vi "Parse MEGA.vi"(10 "path":path) -> (2 "MEGA Traj":T9(array[cluster]) {"?"."Overrides"."Angle Override" step=5.0; "?"."Overrides"."Velocity Override" step=5.0; "?"."Overrides"."Angular Override" step=5.0; "?"."Angular Limits"."Jerk (deg/s^3)" min=0.0 step=1.0; "?"."Angular Limits"."Accel (deg/s^2)" min=0.0; "?"."Angular Limits"."Velocity (deg/s)" min=0.0})   [LabVIEW 2023]
uses:
  Types/Trajectory Data.ctl
  Types/Segment Type.ctl
  Types/Single Cmd Info.ctl
  <vilib>/picture/picture.llb/imagedata.ctl
  Types/Overrides.ctl
  Types/Angluar Limits.ctl
  Types/Drive Type.ctl
  Types/Path Type.ctl
  Types/Availible Command systems for auto.ctl
  Types/Limits.ctl
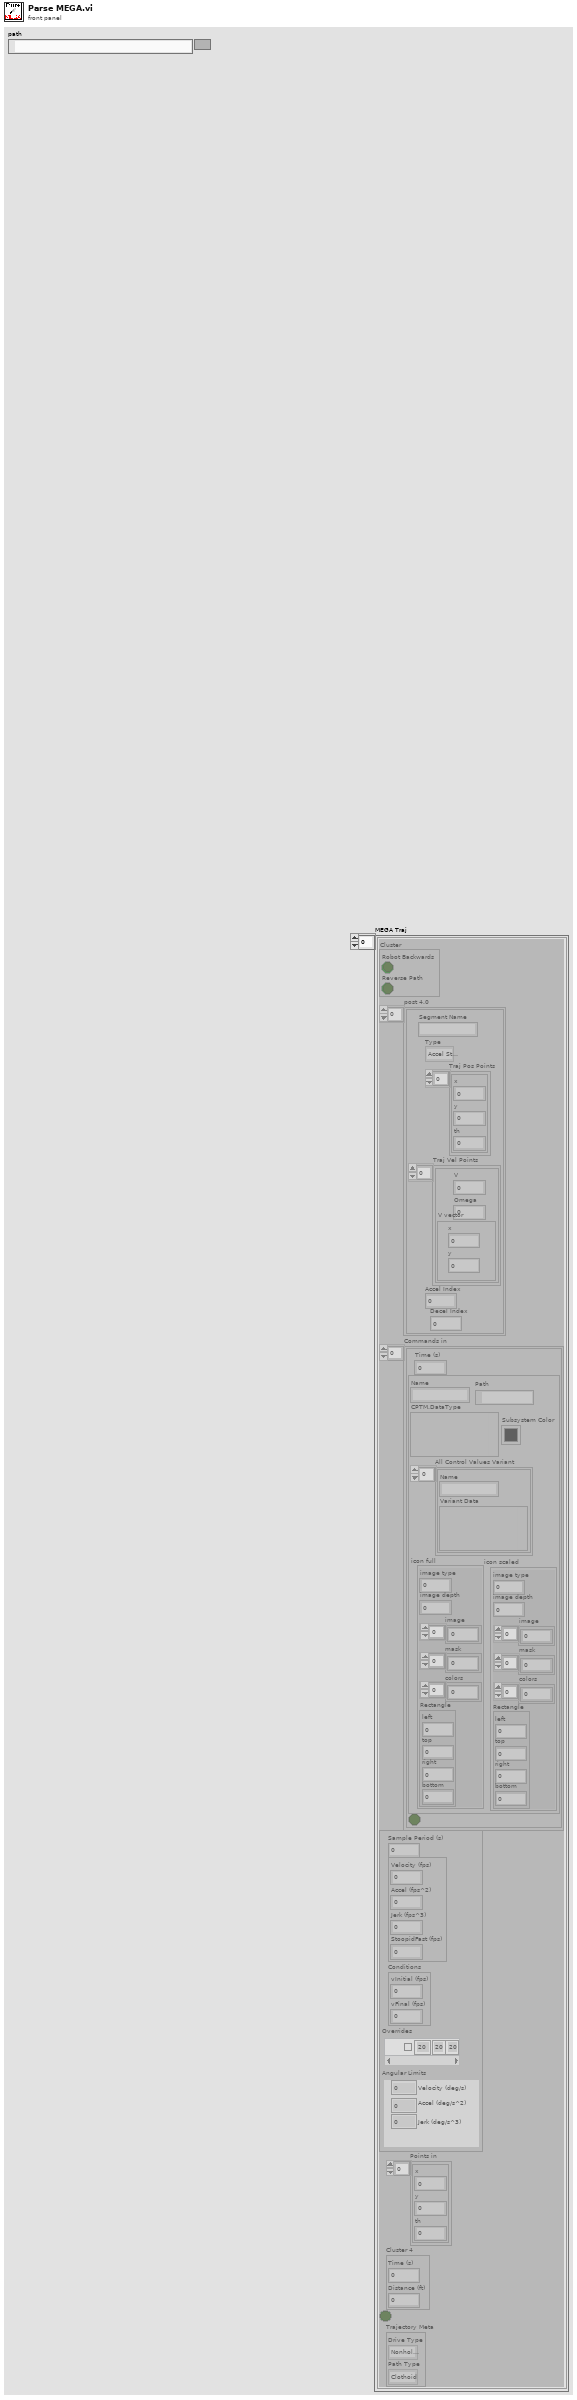
[diagram p1: front panel]
types:
  T1 = typedef "Trajectory Data.ctl" = cluster{"Segment Name":string, "Type":T2, "Traj Pos Points":cluster{"x":dbl, "y":dbl, "th":dbl}[], "Traj Vel Points":cluster{"V":dbl, "Omega":dbl, "V vector":cluster{"y":dbl, "x":dbl}}[], "Accel Index":i32, "Decel Index":i32}[]
  T2 = typedef "Segment Type.ctl" = enum16{"Accel Straight", "Const Straight", "Blend", "Circle", "Bezier"}
  T3 = typedef "Single Cmd Info.ctl" = cluster{"Name":string, "CPTM.DataType":variant, "All Control Values Variant":cluster{"Name":string, "Variant Data":variant}[], "icon full":T4, "icon scaled":T4, "Path":path, "Subsystem Color":u32}
  T4 = typedef "imagedata.ctl" = cluster{"image type":i32, "image depth":i32, "image":u8[], "mask":u8[], "colors":u32[], "Rectangle":cluster{"left":i16, "top":i16, "right":i16, "bottom":i16}}
  T5 = typedef "Overrides.ctl" = cluster{"Count":string, "Angular Override":dbl, "Enabled?":bool, "Velocity Override":dbl, "Angle Override":dbl}[]
  T6 = typedef "Angluar Limits.ctl" = cluster{"Velocity (deg/s)":dbl, "Accel (deg/s^2)":dbl, "Jerk (deg/s^3)":dbl}
  T7 = typedef "Drive Type.ctl" = enum16{"Nonholonomic", "Holonomic"}
  T8 = typedef "Path Type.ctl" = enum16{"Clothoid", "Bezier"}
  T9 = cluster{"Cluster":cluster{"Robot Backwards":bool, "Reverse Path":bool}, "post 4.0":T1, "Commands in":cluster{"Time (s)":dbl, T3, bool}[], cluster{"Sample Period (s)":dbl, cluster{"Velocity (fps)":dbl, "Accel (fps^2)":dbl, "Jerk (fps^3)":dbl, "StoopidFast (fps)":dbl}, "Conditions":cluster{"vInitial (fps)":dbl, "vFinal (fps)":dbl}, "Overrides":T5, "Angular Limits":T6}, "Points in":cluster{"x":dbl, "y":dbl, "th":dbl}[], "Cluster 4":cluster{"Time (s)":dbl, "Distance (ft)":dbl}, bool, "Trajectory Meta":cluster{"Drive Type":T7, "Path Type":T8}}[]
  T10 = cluster{"Segment Name":string, "Type":T2, "Traj Pos Points":cluster{"x":dbl, "y":dbl, "th":dbl}[], "Traj Vel Points":cluster{"V":dbl, "Omega":dbl}[], "Accel Index":i32, "Decel Index":i32}[]
  T11 = cluster{"Sample Period (s)":dbl, "Limits 2":cluster{"Velocity (fps)":dbl, "Acceleration (fps^2)":dbl, "Jerk (fps^3)":dbl}, "Conditions":cluster{"vInitial (fps)":dbl, "vFinal (fps)":dbl}, " Acceleration Overrides":cluster{"Angular \nAccelerations":dbl[], "Accel Override Bools":bool[]}}
  T12 = cluster{"Velocity":dbl, "Sample Time":dbl, "Accel":dbl}
  T13 = cluster{"Sample Period (s)":dbl, "Limits":cluster{"Velocity (fps)":dbl, "Acceleration (fps^2)":dbl, "Jerk (fps^3)":dbl}, "Conditions":cluster{"vInitial (fps)":dbl, "vFinal (fps)":dbl}}
  T14 = cluster{"Sample Period (s)":dbl, "Limits":cluster{"Velocity (fps)":dbl, "Acceleration (fps^2)":dbl, "Jerk (fps^3)":dbl}, "Conditions":cluster{"vInitial (fps)":dbl, "vFinal (fps)":dbl}, "Min Rads":dbl[]}
  T15 = typedef "Availible Command systems for auto.ctl" = u16
  T16 = cluster{"Time into Path":dbl, "System":T15, "Item Selected?":bool, "System Selection":T15}[]
  T17 = cluster{"Sample Period (s)":dbl, "Limits 2":cluster{"Velocity (fps)":dbl, "Acceleration (fps^2)":dbl, "Jerk (fps^3)":dbl, "Stoopid Fast":dbl}, "Conditions":cluster{"vInitial (fps)":dbl, "vFinal (fps)":dbl}, " Acceleration Overrides":cluster{"Angular \nAccelerations":dbl[], "Accel Override Bools":bool[]}}
  T18 = cluster{"Sample Period (s)":dbl, "Limits":cluster{"Velocity (fps)":dbl, "Accel (fps^2)":dbl, "Turn Accel (fps^2)":dbl, "Jerk (fps^3)":dbl}, "Conditions":cluster{"vInitial (fps)":dbl, "vFinal (fps)":dbl}, cluster{dbl[], bool[]}}
  T19 = cluster{"Reverse Path":bool, "Robot Backwards":bool}
  T20 = cluster{"Robot Backwards":bool, "Reverse Path":bool}
  T21 = typedef "Limits.ctl" = cluster{"Velocity (fps)":dbl, "Accel (fps^2)":dbl, "Jerk (fps^3)":dbl, "StoopidFast (fps)":dbl}
  T22 = cluster{"Sample Period (s)":dbl, "Limits":T21, "Conditions":cluster{"vInitial (fps)":dbl, "vFinal (fps)":dbl}, "Overrides":T5, "Angular Limits":T6}
  T23 = cluster{"Velocity":dbl, "Accel":dbl, "Accel":dbl, "Velocity":dbl}
  T24 = cluster{"Velocity (fps)":dbl, "Acceleration (fps^2)":dbl, "Jerk (fps^3)":dbl}
  T25 = cluster{"vInitial (fps)":dbl, "vFinal (fps)":dbl}
  T26 = cluster{"Velocity (fps)":dbl, "Acceleration (fps^2)":dbl, "Jerk (fps^3)":dbl, "Velocity (fps)":dbl}
  T27 = cluster{string, "Angular Multiplier":dbl, bool, "Velocity (fps)":dbl, "Velocity (fps)":dbl}
  T28 = cluster{"Angular \nAccelerations":dbl[], "Accel Override Bools":bool[]}
  T29 = cluster{"Velocity (fps)":dbl, "Acceleration (fps^2)":dbl, "Jerk (fps^3)":dbl, "Stoopid Fast":dbl}
  T30 = cluster{"Velocity (fps)":dbl, "Accel (fps^2)":dbl, "Turn Accel (fps^2)":dbl, "Jerk (fps^3)":dbl}
  T31 = cluster{"Velocity (fps)":dbl, "Accel (fps^2)":dbl, "Jerk (fps^3)":dbl, "StoopidFast (fps)":dbl}
  T32 = cluster{"Sample Period (s)":dbl, cluster{"Velocity (fps)":dbl, "Accel (fps^2)":dbl, "Jerk (fps^3)":dbl, "StoopidFast (fps)":dbl}, "Conditions":cluster{"vInitial (fps)":dbl, "vFinal (fps)":dbl}, "Overrides":T5, "Angular Limits":T6}
  T33 = cluster{"Cluster":cluster{"Robot Backwards":bool, "Reverse Path":bool}, "post 4.0":T1, "Commands in":cluster{"Time (s)":dbl, T3, bool}[], cluster{"Sample Period (s)":dbl, cluster{"Velocity (fps)":dbl, "Accel (fps^2)":dbl, "Jerk (fps^3)":dbl, "StoopidFast (fps)":dbl}, "Conditions":cluster{"vInitial (fps)":dbl, "vFinal (fps)":dbl}, "Overrides":T5, "Angular Limits":T6}, "Points in":cluster{"x":dbl, "y":dbl, "th":dbl}[], "Cluster 4":cluster{"Time (s)":dbl, "Distance (ft)":dbl}, bool, "Trajectory Meta":cluster{"Drive Type":T7, "Path Type":T8}}
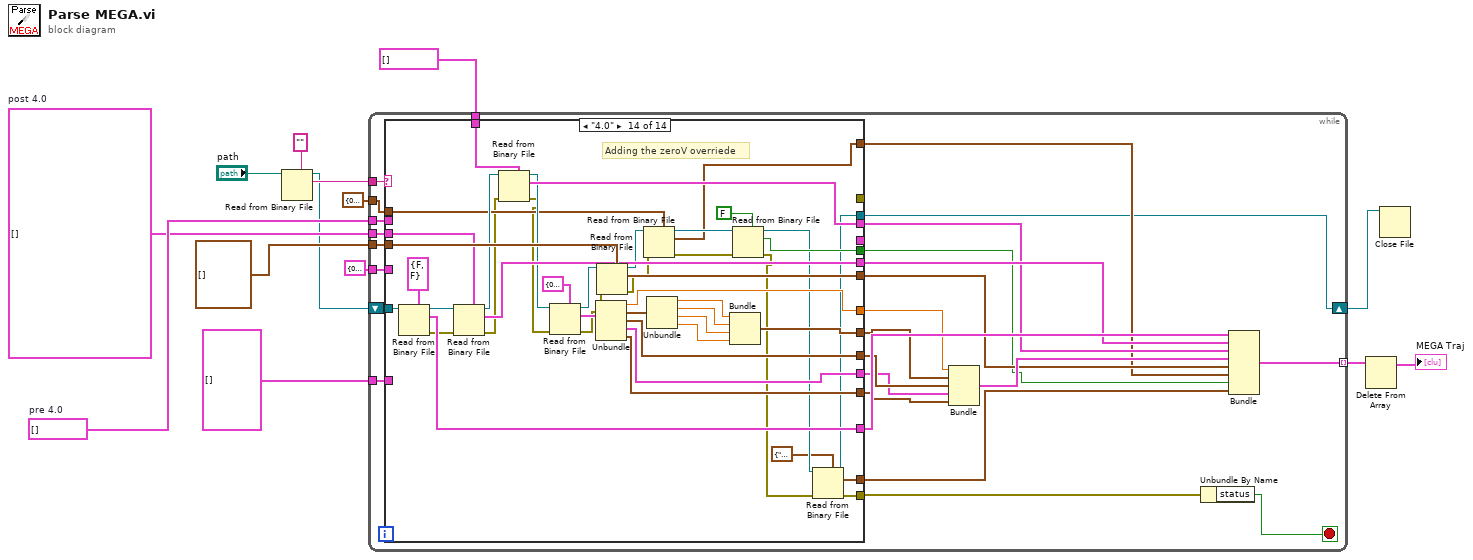
[diagram p0: block diagram]
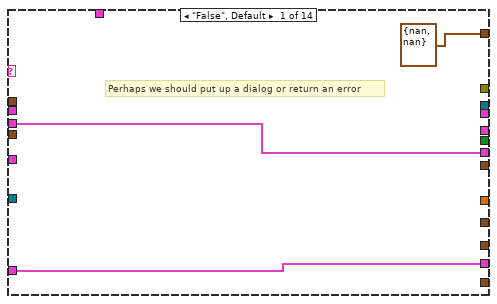
[diagram p2: hidden frame]
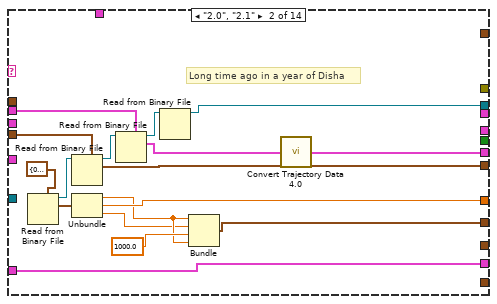
[diagram p3: hidden frame]
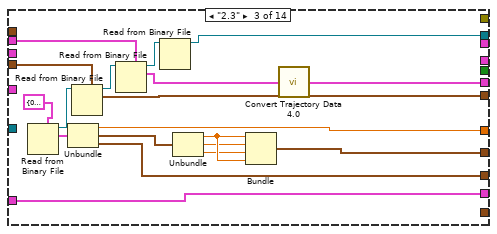
[diagram p4: hidden frame]
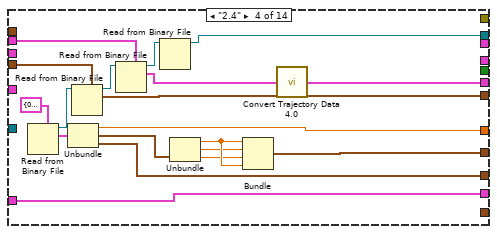
[diagram p5: hidden frame]
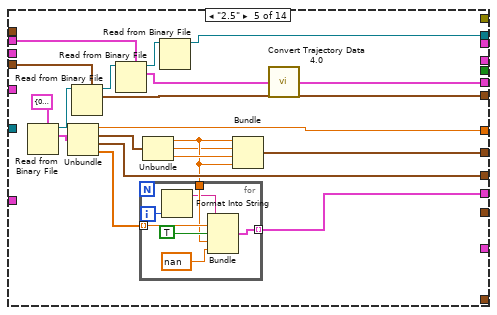
[diagram p6: hidden frame]
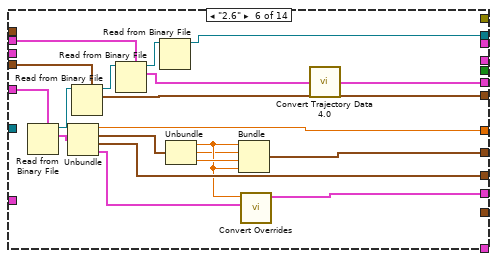
[diagram p7: hidden frame]
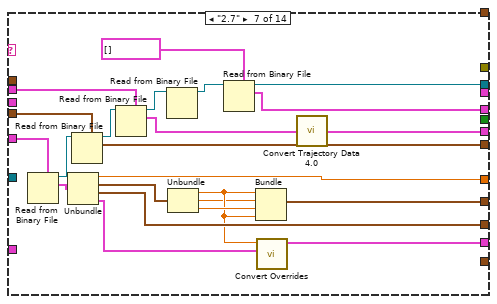
[diagram p8: hidden frame]
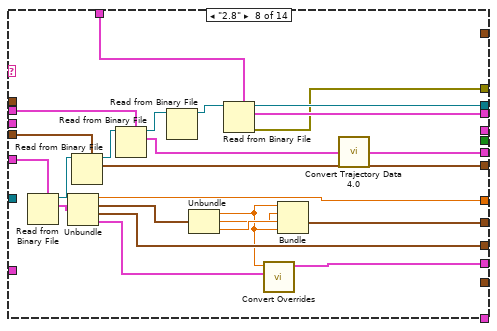
[diagram p9: hidden frame]
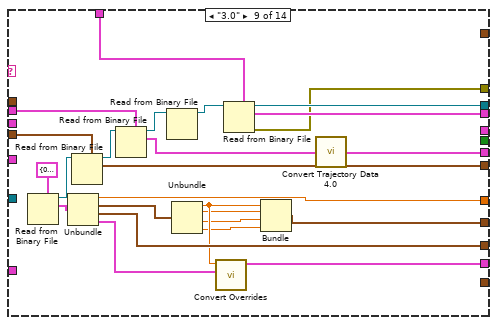
[diagram p10: hidden frame]
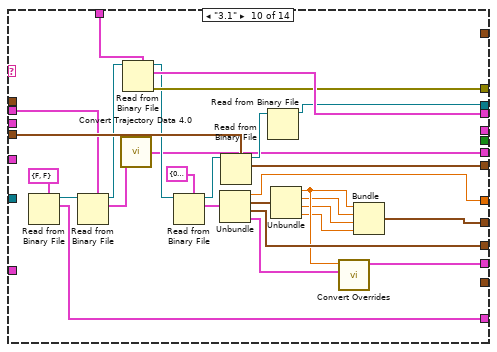
[diagram p11: hidden frame]
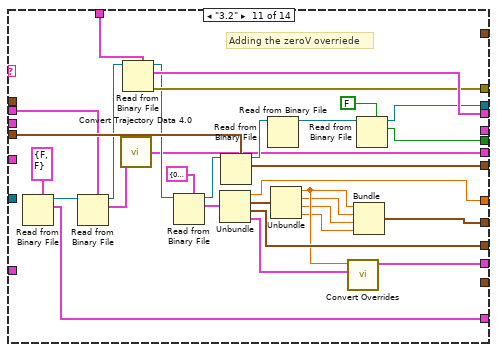
[diagram p12: hidden frame]
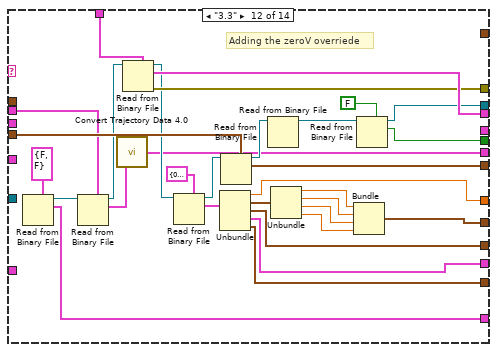
[diagram p13: hidden frame]
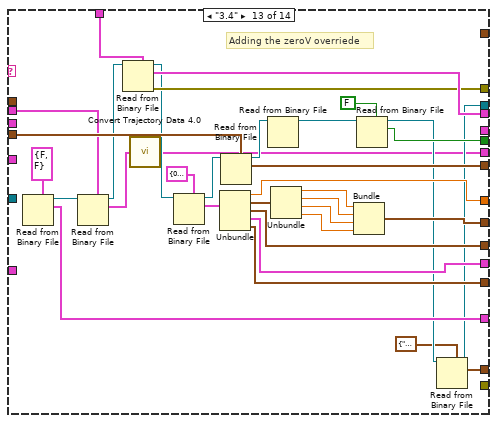
[diagram p14: hidden frame]
diagram:
  w7 = T10 []  # pre 4.0
  w6 = T1 []  # post 4.0
  n1 = Read from Binary File(5:"" ("String"), 11:"path") -> (2:w10:string, 3:w5:refnum<file>)  [unwired: 4 in, 2 out]
  n2 = while {
    tunnel: T11 {"Sample Period (s)"=0.0, "Limits 2"={"Velocity (fps)"=0.0, "Acceleration (fps^2)"=0.0, "Jerk (fps^3)"=0.0}, "Conditions"={"vInitial (fps)"=0.0, "vFinal (fps)"=0.0}, " Acceleration Overrides"={"Angular \nAccelerations"=[], "Accel Override Bools"=[]}} ("Cluster") -> [w40]
    tunnel: cluster{"Time (s)":dbl, T3, bool}[] [] ("Commands in") -> [w39]
    tunnel: cluster{"x":dbl, "y":dbl, "th":dbl}[] [] ("Points in") -> [w38]
    tunnel: w10 -> [w37]
    tunnel: T5 [] ("Overrides") -> [w36]
    tunnel: w7 -> [w35]
    tunnel: w6 -> [w34]
    tunnel: [w20] -> w2 mode=indexing
    tunnel: cluster{"Time (s)":dbl, "Distance (ft)":dbl} {"Time (s)"=0.0, "Distance (ft)"=0.0} ("Cluster 4") -> [w18]
    shift-right: [w16] -> w3
    shift-left: w5 -> [w19]
    stop <- w17 stop-if-true
    n3 = case shown="\"4.0\"" w37 {
      tunnel: w38 -> [_ w58 w77 w96 w116 w143 w166 w190 w215 w243 w274 w305 w339 w382]
      tunnel: [_ w57 w76 w95 w115 w142 w165 w189 w214 w242 w273 w304 w338 w381] -> w29
      tunnel: w35 -> [_ w56 w75 w94 w114 w141 w164 w188 w213 w241 w272 w303 w337 _]
      tunnel: [_ w53 w72 w91 w111 w138 w157 w181 w206 w232 w249 w283 w310 w355] -> w16
      tunnel: [_ w51 w71 w90 w110 w137 w161 w185 w210 w219 w251 w285 w319 w364] -> w25
      tunnel: [_ w47 w65 w83 w104 w132 w151 w176 w194 w224 w256 w290 w324 w369] -> w24
      tunnel: [_ _ w70 w89 w109 w136 w160 w184 w209 w240 w271 w302 w336 w380] -> w23
      tunnel: [w43 w46 w64 w82 w103 w130 w148 w173 w200 w228 w260 w279 w314 w359] -> w22
      tunnel: [w41 w44 w61 w80 w99 w126 w146 w169 w193 w218 w246 w277 w308 w379] -> w31
      tunnel: [_ _ _ _ _ _ w156 _ _ _ _ _ _ _] -> _
      tunnel: w39 -> [_ _ _ _ _ _ _ w180 w205 w238 w269 w300 w334 w378]
      tunnel: [_ _ _ _ _ _ _ w179 w204 w237 w268 w299 w333 w377] -> w30
      tunnel: [_ _ _ _ _ _ _ w178 w203 w236 w267 w298 w332 _] -> _
      tunnel: w40 -> [_ _ _ _ _ w134 w154 w174 _ _ _ _ _ _]
      tunnel: [_ _ _ _ _ _ _ _ _ w227 w259 w292 w326 w371] -> w32
      tunnel: w36 -> [w43 w46 w64 w82 _ _ _ _ _ _ _ _ _ _]
      tunnel: [_ _ _ _ _ _ _ _ _ _ w247 w281 w316 w361] -> w27
      tunnel: [cluster{"Time (s)":dbl, "Distance (ft)":dbl} {"Time (s)"=nan, "Distance (ft)"=nan} ("Cluster 4") _ _ _ _ _ _ _ _ _ _ _ _ w350] -> w28
      tunnel: [_ _ _ _ _ _ _ _ _ _ _ w278 w313 w358] -> w21
      tunnel: [_ _ _ _ _ _ _ _ _ _ _ _ w309 w354] -> w26
      tunnel: w34 -> [w41 _ _ _ _ _ _ _ _ _ _ _ _ w353]
      tunnel: w19 -> [_ _ _ _ _ _ _ _ _ _ _ _ _ w352]
      tunnel: w18 -> [_ _ _ _ _ _ _ _ _ _ _ _ _ w351]
      tunnel: [_ _ _ _ _ _ _ _ _ _ _ _ _ w342] -> w15
      frame "False", Default {
        # "Perhaps we should put up a dialog or return an error"
      }
      frame "2.0", "2.1" {
        # "Long time ago in a year of Disha"
        n4 = Read from Binary File(5:T12 {"Velocity"=0.0, "Sample Time"=0.0, "Accel"=0.0}) -> (2:w60:T12, 3:w59:refnum<file>)  [unwired: 5 in, 2 out]
        n5 = Read from Binary File(5:w58, 11:w59) -> (2:w57:cluster{"x":dbl, "y":dbl, "th":dbl}[], 3:w55:refnum<file>)  [unwired: 4 in, 2 out]
        n6 = Unbundle(w60) -> ("Velocity"=w48:dbl, "Sample Time"=w51:dbl, "Accel"=w45:dbl)
        n7 = Read from Binary File(5:w56, 11:w55) -> (2:w49:T10, 3:w54:refnum<file>)  [unwired: 4 in, 2 out]
        n8 = Read from Binary File(11:w54) -> (3:w53:refnum<file>)  [unwired: 5 in, 3 out]
        n9 = Bundle("Velocity"=w48, "Accel"=w45, "Accel"=1000.0, "Velocity"=w48) -> (w47:T23)  [unwired: 1 in]
        n10 = call "Convert Trajectory Data 4.0.vi"("pre 4.0"=w49) -> ("post 4.0"=w44:T1)
      }
      frame "2.3" {
        n11 = Read from Binary File(5:T13 {"Sample Period (s)"=0.0, "Limits"={"Velocity (fps)"=0.0, "Acceleration (fps^2)"=0.0, "Jerk (fps^3)"=0.0}, "Conditions"={"vInitial (fps)"=0.0, "vFinal (fps)"=0.0}}) -> (2:w79:T13, 3:w78:refnum<file>)  [unwired: 5 in, 2 out]
        n12 = Unbundle(w79) -> ("Sample Period (s)"=w71:dbl, "Limits"=w62:T24, "Conditions"=w70:T25)
        n13 = Read from Binary File(5:w77, 11:w78) -> (2:w76:cluster{"x":dbl, "y":dbl, "th":dbl}[], 3:w74:refnum<file>)  [unwired: 4 in, 2 out]
        n14 = Read from Binary File(5:w75, 11:w74) -> (2:w68:T10, 3:w73:refnum<file>)  [unwired: 4 in, 2 out]
        n15 = Read from Binary File(11:w73) -> (3:w72:refnum<file>)  [unwired: 5 in, 3 out]
        n16 = Unbundle(w62) -> ("Velocity (fps)"=w67:dbl, "Acceleration (fps^2)"=w63:dbl, "Jerk (fps^3)"=w66:dbl)
        n17 = Bundle("Velocity (fps)"=w67, "Acceleration (fps^2)"=w63, "Jerk (fps^3)"=w66, "Velocity (fps)"=w67) -> (w65:T26)  [unwired: 1 in]
        n18 = call "Convert Trajectory Data 4.0.vi"("pre 4.0"=w68) -> ("post 4.0"=w61:T1)
      }
      frame "2.4" {
        n19 = Read from Binary File(5:T13 {"Sample Period (s)"=0.0, "Limits"={"Velocity (fps)"=0.0, "Acceleration (fps^2)"=0.0, "Jerk (fps^3)"=0.0}, "Conditions"={"vInitial (fps)"=0.0, "vFinal (fps)"=0.0}}) -> (2:w98:T13, 3:w97:refnum<file>)  [unwired: 5 in, 2 out]
        n20 = Unbundle(w98) -> ("Sample Period (s)"=w90:dbl, "Limits"=w84:T24, "Conditions"=w89:T25)
        n21 = Read from Binary File(5:w96, 11:w97) -> (2:w95:cluster{"x":dbl, "y":dbl, "th":dbl}[], 3:w93:refnum<file>)  [unwired: 4 in, 2 out]
        n22 = Read from Binary File(5:w94, 11:w93) -> (2:w87:T10, 3:w92:refnum<file>)  [unwired: 4 in, 2 out]
        n23 = Read from Binary File(11:w92) -> (3:w91:refnum<file>)  [unwired: 5 in, 3 out]
        n24 = Unbundle(w84) -> ("Velocity (fps)"=w86:dbl, "Acceleration (fps^2)"=w81:dbl, "Jerk (fps^3)"=w85:dbl)
        n25 = Bundle("Velocity (fps)"=w86, "Acceleration (fps^2)"=w81, "Jerk (fps^3)"=w85, "Velocity (fps)"=w86) -> (w83:T26)  [unwired: 1 in]
        n26 = call "Convert Trajectory Data 4.0.vi"("pre 4.0"=w87) -> ("post 4.0"=w80:T1)
      }
      frame "2.5" {
        n27 = Read from Binary File(5:T14 {"Sample Period (s)"=0.0, "Limits"={"Velocity (fps)"=0.0, "Acceleration (fps^2)"=0.0, "Jerk (fps^3)"=0.0}, "Conditions"={"vInitial (fps)"=0.0, "vFinal (fps)"=0.0}, "Min Rads"=[20.0, 20.0, 20.0, 20.0, 20.0]}) -> (2:w118:T14, 3:w117:refnum<file>)  [unwired: 5 in, 2 out]
        n28 = Unbundle(w118) -> ("Sample Period (s)"=w110:dbl, "Limits"=w105:T24, "Conditions"=w109:T25, "Min Rads"=w102:dbl[])
        n29 = Read from Binary File(5:w116, 11:w117) -> (2:w115:cluster{"x":dbl, "y":dbl, "th":dbl}[], 3:w113:refnum<file>)  [unwired: 4 in, 2 out]
        n30 = Read from Binary File(5:w114, 11:w113) -> (2:w107:T10, 3:w112:refnum<file>)  [unwired: 4 in, 2 out]
        n31 = Unbundle(w105) -> ("Velocity (fps)"=w101:dbl, "Acceleration (fps^2)"=w100:dbl, "Jerk (fps^3)"=w106:dbl)
        n32 = for {
          tunnel: [w124] -> w103 mode=indexing
          tunnel: w102 -> [w123] mode=indexing
          tunnel: w101 -> [w122]
          i -> [w121]
          n33 = Format Into String(w121) -> (resulting string=w120:string)  [unwired: 3 in, 1 out]
          n34 = Bundle(w120, "Angular Multiplier"=w123, TRUE, "Velocity (fps)"=w122, "Velocity (fps)"=nan) -> (w124:T27)  [unwired: 1 in]
        }
        n35 = Read from Binary File(11:w112) -> (3:w111:refnum<file>)  [unwired: 5 in, 3 out]
        n36 = Bundle("Velocity (fps)"=w101, "Acceleration (fps^2)"=w100, "Jerk (fps^3)"=w106, "Velocity (fps)"=w101) -> (w104:T26)  [unwired: 1 in]
        n37 = call "Convert Trajectory Data 4.0.vi"("pre 4.0"=w107) -> ("post 4.0"=w99:T1)
      }
      frame "2.6" {
        n38 = Read from Binary File(5:w134) -> (2:w145:T11, 3:w144:refnum<file>)  [unwired: 5 in, 2 out]
        n39 = Unbundle(w145) -> ("Sample Period (s)"=w137:dbl, "Limits 2"=w131:T24, "Conditions"=w136:T25, "Acceleration Overrides"=w128:T28)
        n40 = Read from Binary File(5:w143, 11:w144) -> (2:w142:cluster{"x":dbl, "y":dbl, "th":dbl}[], 3:w140:refnum<file>)  [unwired: 4 in, 2 out]
        n41 = Read from Binary File(5:w141, 11:w140) -> (2:w135:T10, 3:w139:refnum<file>)  [unwired: 4 in, 2 out]
        n42 = Read from Binary File(11:w139) -> (3:w138:refnum<file>)  [unwired: 5 in, 3 out]
        n43 = Unbundle(w131) -> ("Velocity (fps)"=w129:dbl, "Acceleration (fps^2)"=w127:dbl, "Jerk (fps^3)"=w133:dbl)
        n44 = Bundle("Velocity (fps)"=w129, "Acceleration (fps^2)"=w127, "Jerk (fps^3)"=w133, "Velocity (fps)"=w129) -> (w132:T26)  [unwired: 1 in]
        n45 = call "Convert Overrides.vi"("Cluster"=w128, "Velocity (fps)"=w129) -> ("Overrides"=w130:T5)  [unwired: 9 in]
        n46 = call "Convert Trajectory Data 4.0.vi"("pre 4.0"=w135) -> ("post 4.0"=w126:T1)
      }
      frame "2.7" {
        n47 = Read from Binary File(5:w154) -> (2:w168:T11, 3:w167:refnum<file>)  [unwired: 5 in, 2 out]
        n48 = Unbundle(w168) -> ("Sample Period (s)"=w161:dbl, "Limits 2"=w152:T24, "Conditions"=w160:T25, "Acceleration Overrides"=w149:T28)
        n49 = Read from Binary File(5:w166, 11:w167) -> (2:w165:cluster{"x":dbl, "y":dbl, "th":dbl}[], 3:w163:refnum<file>)  [unwired: 4 in, 2 out]
        n50 = Read from Binary File(5:w164, 11:w163) -> (2:w159:T10, 3:w162:refnum<file>)  [unwired: 4 in, 2 out]
        n51 = Read from Binary File(11:w162) -> (3:w158:refnum<file>)  [unwired: 5 in, 3 out]
        n52 = Unbundle(w152) -> ("Velocity (fps)"=w150:dbl, "Acceleration (fps^2)"=w147:dbl, "Jerk (fps^3)"=w153:dbl)
        n53 = Read from Binary File(5:T16 [] ("Commands"), 11:w158) -> (2:w156:T16, 3:w157:refnum<file>)  [unwired: 4 in, 2 out]
        n54 = Bundle("Velocity (fps)"=w150, "Acceleration (fps^2)"=w147, "Jerk (fps^3)"=w153, "Velocity (fps)"=w150) -> (w151:T26)  [unwired: 1 in]
        n55 = call "Convert Overrides.vi"("Cluster"=w149, "Velocity (fps)"=w150) -> ("Overrides"=w148:T5)  [unwired: 9 in]
        n56 = call "Convert Trajectory Data 4.0.vi"("pre 4.0"=w159) -> ("post 4.0"=w146:T1)
      }
      frame "2.8" {
        n57 = Read from Binary File(5:w174) -> (2:w192:T11, 3:w191:refnum<file>)  [unwired: 5 in, 2 out]
        n58 = Unbundle(w192) -> ("Sample Period (s)"=w185:dbl, "Limits 2"=w177:T24, "Conditions"=w184:T25, "Acceleration Overrides"=w171:T28)
        n59 = Read from Binary File(5:w190, 11:w191) -> (2:w189:cluster{"x":dbl, "y":dbl, "th":dbl}[], 3:w187:refnum<file>)  [unwired: 4 in, 2 out]
        n60 = Read from Binary File(5:w188, 11:w187) -> (2:w183:T10, 3:w186:refnum<file>)  [unwired: 4 in, 2 out]
        n61 = Read from Binary File(11:w186) -> (3:w182:refnum<file>)  [unwired: 5 in, 3 out]
        n62 = Unbundle(w177) -> ("Velocity (fps)"=w172:dbl, "Acceleration (fps^2)"=w170:dbl, "Jerk (fps^3)"=w175:dbl)
        n63 = Read from Binary File(5:w180, 11:w182) -> (0:w178:errorcluster, 2:w179:cluster{"Time (s)":dbl, T3, bool}[], 3:w181:refnum<file>)  [unwired: 4 in, 1 out]
        n64 = call "Convert Overrides.vi"("Cluster"=w171, "Velocity (fps)"=w172) -> ("Overrides"=w173:T5)  [unwired: 9 in]
        n65 = Bundle("Velocity (fps)"=w172, "Acceleration (fps^2)"=w170, "Jerk (fps^3)"=w175, "Velocity (fps)"=w172) -> (w176:T26)  [unwired: 1 in]
        n66 = call "Convert Trajectory Data 4.0.vi"("pre 4.0"=w183) -> ("post 4.0"=w169:T1)
      }
      frame "3.0" {
        n67 = Read from Binary File(5:T17 {"Sample Period (s)"=0.0, "Limits 2"={"Velocity (fps)"=0.0, "Acceleration (fps^2)"=0.0, "Jerk (fps^3)"=0.0, "Stoopid Fast"=0.0}, "Conditions"={"vInitial (fps)"=0.0, "vFinal (fps)"=0.0}, " Acceleration Overrides"={"Angular \nAccelerations"=[], "Accel Override Bools"=[]}} ("Cluster")) -> (2:w217:T17, 3:w216:refnum<file>)  [unwired: 5 in, 2 out]
        n68 = Unbundle(w217) -> ("Sample Period (s)"=w210:dbl, "Limits 2"=w195:T29, "Conditions"=w209:T25, "Acceleration Overrides"=w201:T28)
        n69 = Read from Binary File(5:w215, 11:w216) -> (2:w214:cluster{"x":dbl, "y":dbl, "th":dbl}[], 3:w212:refnum<file>)  [unwired: 4 in, 2 out]
        n70 = Read from Binary File(5:w213, 11:w212) -> (2:w208:T10, 3:w211:refnum<file>)  [unwired: 4 in, 2 out]
        n71 = Read from Binary File(11:w211) -> (3:w207:refnum<file>)  [unwired: 5 in, 3 out]
        n72 = Unbundle(w195) -> ("Velocity (fps)"=w199:dbl, "Acceleration (fps^2)"=w198:dbl, "Jerk (fps^3)"=w197:dbl, "Stoopid Fast"=w196:dbl)
        n73 = call "Convert Overrides.vi"("Cluster"=w201, "Velocity (fps)"=w199) -> ("Overrides"=w200:T5)  [unwired: 9 in]
        n74 = Read from Binary File(5:w205, 11:w207) -> (0:w203:errorcluster, 2:w204:cluster{"Time (s)":dbl, T3, bool}[], 3:w206:refnum<file>)  [unwired: 4 in, 1 out]
        n75 = Bundle("Velocity (fps)"=w199, "Acceleration (fps^2)"=w198, "Jerk (fps^3)"=w197, "Stoopid Fast"=w196) -> (w194:T29)  [unwired: 1 in]
        n76 = call "Convert Trajectory Data 4.0.vi"("pre 4.0"=w208) -> ("post 4.0"=w193:T1)
      }
      frame "3.1" {
        n77 = Read from Binary File(5:T19 {"Reverse Path"=FALSE, "Robot Backwards"=FALSE} ("Cluster")) -> (2:w227:T19, 3:w233:refnum<file>)  [unwired: 5 in, 2 out]
        n78 = Read from Binary File(5:w241, 11:w233) -> (2:w239:T10, 3:w231:refnum<file>)  [unwired: 4 in, 2 out]
        n79 = call "Convert Trajectory Data 4.0.vi"("pre 4.0"=w239) -> ("post 4.0"=w218:T1)
        n80 = Read from Binary File(5:w238, 11:w231) -> (0:w236:errorcluster, 2:w237:cluster{"Time (s)":dbl, T3, bool}[], 3:w230:refnum<file>)  [unwired: 4 in, 1 out]
        n81 = Read from Binary File(5:T18 {"Sample Period (s)"=0.0, "Limits"={"Velocity (fps)"=0.0, "Accel (fps^2)"=0.0, "Turn Accel (fps^2)"=15.0, "Jerk (fps^3)"=0.0}, "Conditions"={"vInitial (fps)"=0.0, "vFinal (fps)"=0.0}, {[], []}} ("Cluster 2"), 11:w230) -> (2:w245:T18, 3:w244:refnum<file>)  [unwired: 4 in, 2 out]
        n82 = Unbundle(w245) -> ("Sample Period (s)"=w219:dbl, "Limits"=w226:T30, "Conditions"=w240:T25, w229:cluster{dbl[], bool[]})
        n83 = Read from Binary File(5:w243, 11:w244) -> (2:w242:cluster{"x":dbl, "y":dbl, "th":dbl}[], 3:w234:refnum<file>)  [unwired: 4 in, 2 out]
        n84 = Read from Binary File(11:w234) -> (3:w232:refnum<file>)  [unwired: 5 in, 3 out]
        n85 = Unbundle(w226) -> ("Velocity (fps)"=w223:dbl, "Accel (fps^2)"=w222:dbl, "Turn Accel (fps^2)"=w221:dbl, "Jerk (fps^3)"=w220:dbl)
        n86 = call "Convert Overrides.vi"("Cluster"=w229, "Velocity (fps)"=w223) -> ("Overrides"=w228:T5)  [unwired: 9 in]
        n87 = Bundle("Velocity (fps)"=w223, "Accel (fps^2)"=w222, "Turn Accel (fps^2)"=w221, "Jerk (fps^3)"=w220) -> (w224:T30)  [unwired: 1 in]
      }
      frame "3.2" {
        # "Adding the zeroV overriede"
        n88 = Read from Binary File(5:T20 {"Robot Backwards"=FALSE, "Reverse Path"=FALSE} ("Cluster")) -> (2:w259:T20, 3:w264:refnum<file>)  [unwired: 5 in, 2 out]
        n89 = Read from Binary File(5:w272, 11:w264) -> (2:w270:T10, 3:w263:refnum<file>)  [unwired: 4 in, 2 out]
        n90 = call "Convert Trajectory Data 4.0.vi"("pre 4.0"=w270) -> ("post 4.0"=w246:T1)
        n91 = Read from Binary File(5:w269, 11:w263) -> (0:w267:errorcluster, 2:w268:cluster{"Time (s)":dbl, T3, bool}[], 3:w262:refnum<file>)  [unwired: 4 in, 1 out]
        n92 = Read from Binary File(5:T18 {"Sample Period (s)"=0.0, "Limits"={"Velocity (fps)"=0.0, "Accel (fps^2)"=0.0, "Turn Accel (fps^2)"=15.0, "Jerk (fps^3)"=0.0}, "Conditions"={"vInitial (fps)"=0.0, "vFinal (fps)"=0.0}, {[], []}} ("Cluster 2"), 11:w262) -> (2:w276:T18, 3:w275:refnum<file>)  [unwired: 4 in, 2 out]
        n93 = Unbundle(w276) -> ("Sample Period (s)"=w251:dbl, "Limits"=w258:T30, "Conditions"=w271:T25, w261:cluster{dbl[], bool[]})
        n94 = Read from Binary File(5:w274, 11:w275) -> (2:w273:cluster{"x":dbl, "y":dbl, "th":dbl}[], 3:w265:refnum<file>)  [unwired: 4 in, 2 out]
        n95 = Read from Binary File(11:w265) -> (3:w250:refnum<file>)  [unwired: 5 in, 3 out]
        n96 = Unbundle(w258) -> ("Velocity (fps)"=w255:dbl, "Accel (fps^2)"=w254:dbl, "Turn Accel (fps^2)"=w253:dbl, "Jerk (fps^3)"=w252:dbl)
        n97 = call "Convert Overrides.vi"("Cluster"=w261, "Velocity (fps)"=w255) -> ("Overrides"=w260:T5)  [unwired: 9 in]
        n98 = Bundle("Velocity (fps)"=w255, "Accel (fps^2)"=w254, "Turn Accel (fps^2)"=w253, "Jerk (fps^3)"=w252) -> (w256:T30)  [unwired: 1 in]
        n99 = Read from Binary File(5:FALSE, 11:w250) -> (2:w247:bool, 3:w249:refnum<file>)  [unwired: 4 in, 2 out]
      }
      frame "3.3" {
        # "Adding the zeroV overriede"
        n100 = Read from Binary File(5:T20 {"Robot Backwards"=FALSE, "Reverse Path"=FALSE} ("Cluster")) -> (2:w292:T20, 3:w295:refnum<file>)  [unwired: 5 in, 2 out]
        n101 = Read from Binary File(5:w303, 11:w295) -> (2:w301:T10, 3:w294:refnum<file>)  [unwired: 4 in, 2 out]
        n102 = call "Convert Trajectory Data 4.0.vi"("pre 4.0"=w301) -> ("post 4.0"=w277:T1)
        n103 = Read from Binary File(5:w300, 11:w294) -> (0:w298:errorcluster, 2:w299:cluster{"Time (s)":dbl, T3, bool}[], 3:w293:refnum<file>)  [unwired: 4 in, 1 out]
        n104 = Read from Binary File(5:T22 {"Sample Period (s)"=0.0, "Limits"={"Velocity (fps)"=0.0, "Accel (fps^2)"=0.0, "Jerk (fps^3)"=0.0, "StoopidFast (fps)"=0.0}, "Conditions"={"vInitial (fps)"=0.0, "vFinal (fps)"=0.0}, "Overrides"=[], "Angular Limits"={"Velocity (deg/s)"=0.0, "Accel (deg/s^2)"=0.0, "Jerk (deg/s^3)"=0.0}} ("output cluster"), 11:w293) -> (2:w307:T22, 3:w306:refnum<file>)  [unwired: 4 in, 2 out]
        n105 = Unbundle(w307) -> ("Sample Period (s)"=w285:dbl, "Limits"=w291:T21, "Conditions"=w302:T25, "Overrides"=w279:T5, "Angular Limits"=w278:T6)
        n106 = Read from Binary File(5:w305, 11:w306) -> (2:w304:cluster{"x":dbl, "y":dbl, "th":dbl}[], 3:w296:refnum<file>)  [unwired: 4 in, 2 out]
        n107 = Read from Binary File(11:w296) -> (3:w284:refnum<file>)  [unwired: 5 in, 3 out]
        n108 = Unbundle(w291) -> ("Velocity (fps)"=w289:dbl, "Accel (fps^2)"=w288:dbl, "Jerk (fps^3)"=w287:dbl, "StoopidFast (fps)"=w286:dbl)
        n109 = Bundle("Velocity (fps)"=w289, "Accel (fps^2)"=w288, "Jerk (fps^3)"=w287, "StoopidFast (fps)"=w286) -> (w290:T31)  [unwired: 1 in]
        n110 = Read from Binary File(5:FALSE, 11:w284) -> (2:w281:bool, 3:w283:refnum<file>)  [unwired: 4 in, 2 out]
      }
      frame "3.4" {
        # "Adding the zeroV overriede"
        n111 = Read from Binary File(5:T20 {"Robot Backwards"=FALSE, "Reverse Path"=FALSE} ("Cluster")) -> (2:w326:T20, 3:w329:refnum<file>)  [unwired: 5 in, 2 out]
        n112 = Read from Binary File(5:w337, 11:w329) -> (2:w335:T10, 3:w328:refnum<file>)  [unwired: 4 in, 2 out]
        n113 = Read from Binary File(5:w334, 11:w328) -> (0:w332:errorcluster, 2:w333:cluster{"Time (s)":dbl, T3, bool}[], 3:w327:refnum<file>)  [unwired: 4 in, 1 out]
        n114 = call "Convert Trajectory Data 4.0.vi"("pre 4.0"=w335) -> ("post 4.0"=w308:T1)
        n115 = Read from Binary File(5:T22 {"Sample Period (s)"=0.0, "Limits"={"Velocity (fps)"=0.0, "Accel (fps^2)"=0.0, "Jerk (fps^3)"=0.0, "StoopidFast (fps)"=0.0}, "Conditions"={"vInitial (fps)"=0.0, "vFinal (fps)"=0.0}, "Overrides"=[], "Angular Limits"={"Velocity (deg/s)"=0.0, "Accel (deg/s^2)"=0.0, "Jerk (deg/s^3)"=0.0}} ("output cluster"), 11:w327) -> (2:w341:T22, 3:w340:refnum<file>)  [unwired: 4 in, 2 out]
        n116 = Unbundle(w341) -> ("Sample Period (s)"=w319:dbl, "Limits"=w325:T21, "Conditions"=w336:T25, "Overrides"=w314:T5, "Angular Limits"=w313:T6)
        n117 = Read from Binary File(5:w339, 11:w340) -> (2:w338:cluster{"x":dbl, "y":dbl, "th":dbl}[], 3:w330:refnum<file>)  [unwired: 4 in, 2 out]
        n118 = Read from Binary File(11:w330) -> (3:w318:refnum<file>)  [unwired: 5 in, 3 out]
        n119 = Unbundle(w325) -> ("Velocity (fps)"=w323:dbl, "Accel (fps^2)"=w322:dbl, "Jerk (fps^3)"=w321:dbl, "StoopidFast (fps)"=w320:dbl)
        n120 = Bundle("Velocity (fps)"=w323, "Accel (fps^2)"=w322, "Jerk (fps^3)"=w321, "StoopidFast (fps)"=w320) -> (w324:T31)  [unwired: 1 in]
        n121 = Read from Binary File(5:FALSE, 11:w318) -> (2:w316:bool, 3:w312:refnum<file>)  [unwired: 4 in, 2 out]
        n122 = Read from Binary File(5:cluster{"Drive Type":T7, "Path Type":T8} {"Drive Type"=enum."Nonholonomic", "Path Type"=enum."Clothoid"} ("Trajectory Meta"), 11:w312) -> (2:w309:cluster{"Drive Type":T7, "Path Type":T8}, 3:w310:refnum<file>)  [unwired: 4 in, 2 out]
      }
      frame "4.0" {
        # "Adding the zeroV overriede"
        n123 = Read from Binary File(5:T20 {"Robot Backwards"=FALSE, "Reverse Path"=FALSE} ("Cluster"), 11:w352) -> (0:w349:errorcluster, 2:w371:T20, 3:w374:refnum<file>)  [unwired: 4 in, 1 out]
        n124 = Read from Binary File(5:w353, 8:w349, 11:w374) -> (0:w348:errorcluster, 2:w379:T1, 3:w373:refnum<file>)  [unwired: 3 in, 1 out]
        n125 = Read from Binary File(5:w378, 8:w348, 11:w373) -> (0:w347:errorcluster, 2:w377:cluster{"Time (s)":dbl, T3, bool}[], 3:w372:refnum<file>)  [unwired: 3 in, 1 out]
        n126 = Read from Binary File(5:T22 {"Sample Period (s)"=0.0, "Limits"={"Velocity (fps)"=0.0, "Accel (fps^2)"=0.0, "Jerk (fps^3)"=0.0, "StoopidFast (fps)"=0.0}, "Conditions"={"vInitial (fps)"=0.0, "vFinal (fps)"=0.0}, "Overrides"=[], "Angular Limits"={"Velocity (deg/s)"=0.0, "Accel (deg/s^2)"=0.0, "Jerk (deg/s^3)"=0.0}} ("output cluster"), 8:w347, 11:w372) -> (0:w346:errorcluster, 2:w384:T22, 3:w383:refnum<file>)  [unwired: 3 in, 1 out]
        n127 = Unbundle(w384) -> ("Sample Period (s)"=w364:dbl, "Limits"=w370:T21, "Conditions"=w380:T25, "Overrides"=w359:T5, "Angular Limits"=w358:T6)
        n128 = Read from Binary File(5:w382, 8:w346, 11:w383) -> (0:w345:errorcluster, 2:w381:cluster{"x":dbl, "y":dbl, "th":dbl}[], 3:w375:refnum<file>)  [unwired: 3 in, 1 out]
        n129 = Read from Binary File(5:w351, 8:w345, 11:w375) -> (0:w344:errorcluster, 2:w350:cluster{"Time (s)":dbl, "Distance (ft)":dbl}, 3:w363:refnum<file>)  [unwired: 3 in, 1 out]
        n130 = Unbundle(w370) -> ("Velocity (fps)"=w368:dbl, "Accel (fps^2)"=w367:dbl, "Jerk (fps^3)"=w366:dbl, "StoopidFast (fps)"=w365:dbl)
        n131 = Bundle("Velocity (fps)"=w368, "Accel (fps^2)"=w367, "Jerk (fps^3)"=w366, "StoopidFast (fps)"=w365) -> (w369:T31)  [unwired: 1 in]
        n132 = Read from Binary File(5:FALSE, 8:w344, 11:w363) -> (0:w343:errorcluster, 2:w361:bool, 3:w357:refnum<file>)  [unwired: 3 in, 1 out]
        n133 = Read from Binary File(5:cluster{"Drive Type":T7, "Path Type":T8} {"Drive Type"=enum."Nonholonomic", "Path Type"=enum."Clothoid"} ("Trajectory Meta"), 8:w343, 11:w357) -> (0:w342:errorcluster, 2:w354:cluster{"Drive Type":T7, "Path Type":T8}, 3:w355:refnum<file>)  [unwired: 3 in, 1 out]
      }
    }
    n134 = Bundle("Sample Period (s)"=w25, w24, "Conditions"=w23, "Overrides"=w22, "Angular Limits"=w21) -> (w33:T32)  [unwired: 1 in]
    n135 = Unbundle By Name(w15) -> ("status"=w17:bool)
    n136 = Bundle("Cluster"=w32, "post 4.0"=w31, "Commands in"=w30, w33, "Points in"=w29, "Cluster 4"=w28, w27, "Trajectory Meta"=w26) -> (w20:T33)  [unwired: 1 in]
  }
  n137 = Delete From Array(array=w2) -> (array with subset deleted=→"MEGA Traj":T9)  [unwired: 2 in, 1 out]
  n138 = Close File(refnum=w3) -> ()  [unwired: 1 in, 2 out]
